vi "vel calc C0 (express VI) - with Reset.vi"(8 "error in":errorcluster, 9 "Encoder accuracy multiplier":dbl=1.0, 10 "dt in (ms)":i32=-1, 11 "Reinitialise":bool) -> (0 "error out":errorcluster, 1 "dt out (ms)":i32, 2 "dx":dbl, 3 "dx/dt":dbl, 5 "Counter Value":dbl)   [LabVIEW 2017]
uses:
  <vilib>/myRIO/Common/Instrument Driver Framework/myRIO v1.0/Encoder/typedefs/Encoder Signal Mode.ctl
  <vilib>/myRIO/Instrument Drivers/Onboard IO/Encoder/typedefs/Encoder Reference.ctl
  <vilib>/myRIO/Common/Instrument Driver Framework/Utilities/typedefs/myRIO Generic Hardware Reference.ctl
  <vilib>/myRIO/Common/Instrument Driver Framework/Utilities/typedefs/Hardware Version Enum.ctl
  <vilib>/myRIO/Common/Instrument Driver Framework/Utilities/typedefs/myRIO v1.0 Reference.ctl
  <vilib>/myRIO/Common/Instrument Driver Framework/Utilities/typedefs/Generic FPGA Reference.ctl
  <vilib>/myRIO/Common/Instrument Driver Framework/myRIO v1.0/Encoder/typedefs/Encoder Channels Enum.ctl
  <vilib>/myRIO/Common/Instrument Driver Framework/myRIO v1.0/Encoder/typedefs/Encoder Configuration v1.0.ctl
  <vilib>/userdefined/High Color/nirio_resource_hc.ctl
  <vilib>/myRIO/Common/Instrument Driver Framework/Utilities/vis/Is FPGA Ref Available.vi
  <vilib>/myRIO/Common/Instrument Driver Framework/myRIO v1.0/Encoder/vis/myRIO v1.1 Open Encoder.vi
  <vilib>/myRIO/Instrument Drivers/Onboard IO/Encoder/vis/Read.vi
  <vilib>/myRIO/Common/Instrument Driver Framework/Utilities/vis/Validate Channels.vi
  <vilib>/myRIO/Common/Instrument Driver Framework/myRIO v1.0/Encoder/vis/myRIO v1.0 Reserve Encoder.vi
  <vilib>/myRIO/Common/Instrument Driver Framework/myRIO v1.0/Encoder/vis/myRIO v1.0 Build MUX Configuration Encoder.vi
  <vilib>/myRIO/Common/Instrument Driver Framework/myRIO v1.0/Resource Manager/vis/myRIO v1.0 Reserve Channel List.vi
  <vilib>/myRIO/Common/Instrument Driver Framework/myRIO v1.0/Resource Manager/vis/myRIO v1.0 Create Configuration List.vi
  <vilib>/myRIO/Common/Instrument Driver Framework/myRIO v1.0/Resource Manager/vis/myRIO v1.0 Reserve Channel.vi
  <vilib>/myRIO/Common/Instrument Driver Framework/myRIO v1.0/Resource Manager/vis/myRIO v1.0 Unreserve Channel.vi
  <vilib>/myRIO/Common/Instrument Driver Framework/myRIO v1.0/Resource Manager/vis/myRIO v1.0 Build Mutex Name.vi
  <vilib>/Utility/VariantDataType/GetNumericInfo.vi
  <vilib>/Utility/error.llb/Error Cluster From Error Code.vi
  <vilib>/myRIO/Common/Instrument Driver Framework/myRIO v1.0/myRIO v1.1 Open.vi
  <vilib>/myRIO/Common/Instrument Driver Framework/Utilities/vis/IO Manager.vi
  <vilib>/myRIO/Common/Instrument Driver Framework/Utilities/vis/Configuration Manager.vi
  <vilib>/myRIO/Common/Instrument Driver Framework/myRIO v1.0/Resource Manager/vis/myRIO v1.0 Configure IO.vi
  <vilib>/myRIO/Common/Instrument Driver Framework/myRIO v1.0/myRIO v1.0 Close.vi
  <vilib>/myRIO/Common/Instrument Driver Framework/myRIO v1.0/Encoder/vis/myRIO v1.0 Configure Encoder.vi
  <vilib>/myRIO/Common/Instrument Driver Framework/myRIO v1.0/Encoder/vis/myRIO v1.0 Read Encoder.vi
  <vilib>/myRIO/Express VI/Onboard IO/Encoder/Encoder Express VI.xnode
  <vilib>/myRIO/Instrument Drivers/Onboard IO/Encoder/vis/myRIO Encoder Open.xnode
  <vilib>/myRIO/Common/Instrument Driver Framework/myRIO v1.0/Encoder/typedefs/Encoder Count Direction Enum.ctl
  <vilib>/myRIO/Instrument Drivers/Onboard IO/Encoder/Encoder.lvlib
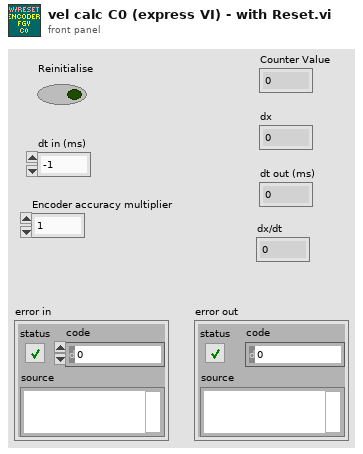
[diagram p1: front panel]
types:
  T1 = typedef "Encoder.lvlib/Encoder Reference.ctl" = cluster{"myRIO Reference":T2, "Encoder Channels Enum":T6}
  T2 = typedef "myRIO Generic Hardware Reference.ctl" = cluster{"myRIO Model":T3, "myRIO Hardware Reference":T4}
  T3 = typedef "Hardware Version Enum.ctl" = enum16{"Unknown", "myRIO-1900", "myRIO-1950", "roboRIO", "NI ELVIS RIO CM"}
  T4 = typedef "myRIO v1.0 Reference.ctl" = cluster{"Generic FPGA Reference":T5, "Allow multiple opens":bool}
  T5 = typedef "Generic FPGA Reference.ctl" = refnum<k20>
  T6 = typedef "Encoder Channels Enum.ctl" = enum16{"Not Connected", "C/ENC0", "C/ENC1", "A/ENC", "B/ENC", "DIO/ENC0", "DIO/ENC1", "DIO/ENC2", "DIO/ENC3", "DIO/ENC4"}
  T7 = typedef "Encoder Signal Mode.ctl" = enum16{"Quadrature phase signal", "Step and direction signal"}
  T8 = typedef "nirio_resource_hc.ctl" = tag
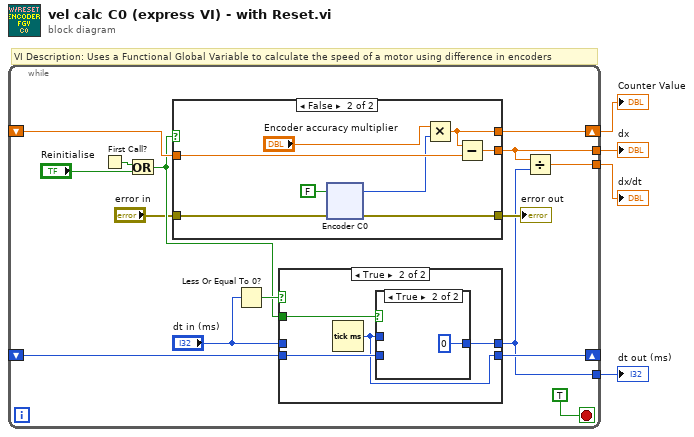
[diagram p0: block diagram]
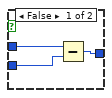
[diagram p3: hidden frame]
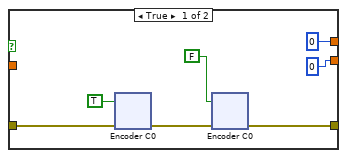
[diagram p4: hidden frame]
diagram:
  # "VI Description: Uses a Functional Global Variable to calculate the speed of a motor using difference in encoders"
  n1 = while {
    shift-right: [w17] -> w3
    shift-left: _ -> [w18]
    tunnel: [w16] -> w4
    tunnel: [w15] -> w2
    shift-right: [w10] -> _
    shift-left: _ -> [w9]
    tunnel: [w5] -> w1
    stop <- TRUE stop-if-true
    n2 = First Call?() -> (First Call?: T/F=w13:bool)
    n3 = Or(x=w13, y="Reinitialise") -> (x .or. y?=w11:bool)
    n4 = case shown="False" w11 {
      tunnel: w18 -> [_ w136]
      tunnel: [0 ("Counter Value") w129] -> w17
      tunnel: [0 w135] -> w16
      tunnel: "error in" -> [w31 w133]
      tunnel: [w30 w132] -> w7
      frame True {
        n5 = xnode "Encoder C0"("error in (no error)"=w31, "Reset Counter"=TRUE) -> ("error out"=w33:errorcluster)  [unwired: 3 out]
        n6 = xnode "Encoder C0"("error in (no error)"=w33, "Reset Counter"=FALSE) -> ("error out"=w30:errorcluster)  [unwired: 3 out]
      }
      frame False {
        n7 = xnode "Encoder C0"("error in (no error)"=w133, "Reset Counter"=FALSE) -> ("error out"=w132:errorcluster, "Counter Value"=w131:i32)  [unwired: 2 out]
        n8 = Multiply(x="Encoder accuracy multiplier", y=w131) -> (x*y=w129:dbl)
        n9 = Subtract(x=w129, y=w136) -> (x-y=w135:dbl)
      }
    }
    "error out" <- w7
    n10 = Less Or Equal To 0?(x="dt in (ms)") -> (x <= 0?=w14:bool)
    n11 = case shown="True" w14 {
      tunnel: w9 -> [w21 w25]
      tunnel: [w21 w24] -> w10
      tunnel: w11 -> [_ w23]
      tunnel: [w20 w22] -> w5
      tunnel: "dt in (ms)" -> [w20 _]
      frame False {
      }
      frame True {
        n12 = Tick Count (ms)() -> (millisecond timer value=w24:u32)
        n13 = case shown="True" w23 {
          tunnel: [w28 u32 0] -> w22
          tunnel: w25 -> [w27 _]
          tunnel: w24 -> [w26 _]
          frame False {
            n14 = Subtract(x=w26, y=w27) -> (x-y=w28:u32)
          }
          frame True {
          }
        }
      }
    }
    n15 = Divide(x=w16, y=w5) -> (x/y=w15:dbl)
  }
  "Counter Value" <- w3
  "dx" <- w4
  "dt out (ms)" <- w1
  "dx/dt" <- w2
